vi "dfd_NStage Calculate CIC Filter Parameters.vi"(6 "fs [Hz]":dbl=4.0, 8 "error in (no error)":errorcluster, 10 "freq spec":T1, 11 "CIC factor":i32=5) -> (0 "error out":errorcluster, 1 "shaping para":cluster{"fpass":dbl, "stop":dbl}, 2 "masking para":cluster{"fpass":dbl, "fstop":dbl}, 3 "CIC fstop":dbl)   [LabVIEW 2017, in "NI_DigFilterLicensed.lvlib"]
uses:
  <vilib>/addons/Digital Filter Design/NI_DigFilterLicensed.lvlib
  <vilib>/addons/Digital Filter Design/_Objects.llb/DFD Multirate Filter Specification (Design).ctl
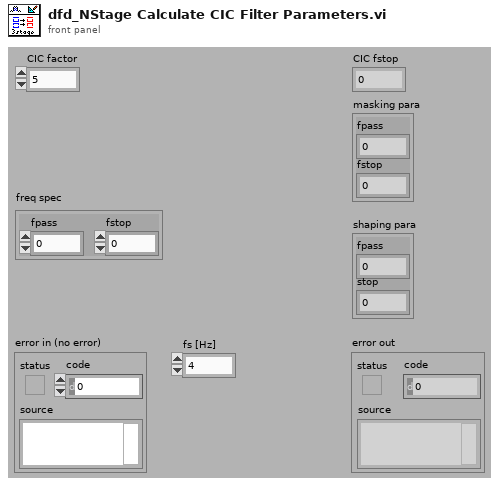
[diagram p1: front panel]
types:
  T1 = typedef "NI_DigFilterLicensed.lvlib/DFD Multirate Filter Specification (Design).ctl" = cluster{"fpass":dbl, "fstop":dbl}
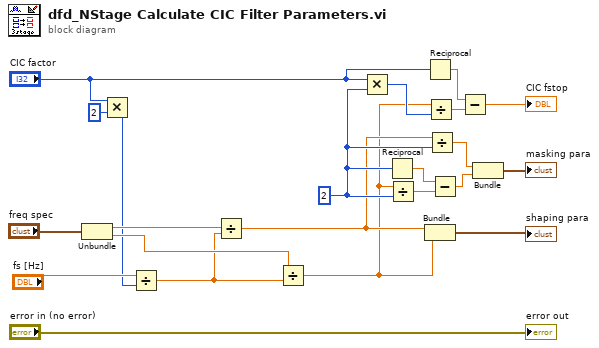
[diagram p0: block diagram]
diagram:
  w13 = 2 ("second factor")
  n1 = Unbundle("freq spec") -> ("fpass"=w10:dbl, "fstop"=w8:dbl)
  n2 = Multiply(x="CIC factor", y=2) -> (x*y=w2:i32)
  n3 = Divide(x="fs [Hz]", y=w2) -> (x/y=w1:dbl)
  n4 = Divide(x=w10, y=w1) -> (x/y=w9:dbl)
  n5 = Divide(x=w8, y=w1) -> (x/y=w7:dbl)
  n6 = Multiply(x="CIC factor", y=w13) -> (x*y=w14:i32)
  n7 = Reciprocal(x=w13) -> (1/x=w21:dbl)
  n8 = Divide(x=w7, y=w13) -> (x/y=w20:dbl)
  n9 = Reciprocal(x="CIC factor") -> (1/x=w16:dbl)
  n10 = Bundle(w9, w7) -> (→"shaping para":cluster{dbl, dbl})  [unwired: 1 out]
  n11 = Divide(x=w7, y=w14) -> (x/y=w15:dbl)
  n12 = Divide(x=w9, y=w13) -> (x/y=w18:dbl)
  n13 = Subtract(x=w21, y=w20) -> (x-y=w17:dbl)
  n14 = Subtract(x=w16, y=w15) -> (x-y=→"CIC fstop":dbl)
  n15 = Bundle(w18, w17) -> (→"masking para":cluster{dbl, dbl})  [unwired: 1 out]
  "error out" <- "error in (no error)"
